vi "Move.vi"(0 "FSM.Edge in":refnum<class "FSM.Edge.lvclass">, 9 "delta":cluster{"X":dbl, "Y":dbl}) -> (4 "FSM.Edge out":refnum<class "FSM.Edge.lvclass">)   [LabVIEW 2020, in "FSM.Edge.lvclass"]
uses:
  FSM.Edge.lvclass
  FSM.Edge.lvclass/FSM.Edge.ctl
  FSM.Label/FSM.Label.lvclass
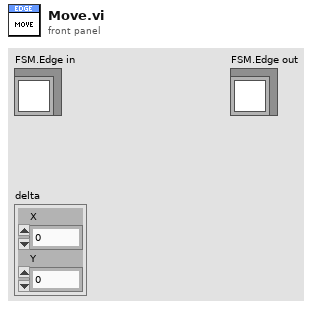
[diagram p1: front panel]
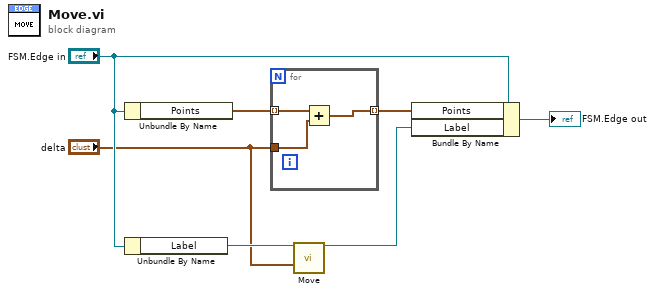
[diagram p0: block diagram]
diagram:
  n1 = Unbundle By Name("FSM.Edge in") -> ("Points"=w2:cluster{"x":i16, "y":i16}[])
  n2 = Unbundle By Name("FSM.Edge in") -> ("Label"=w4:refnum<class "FSM.Label.lvclass">)
  n3 = for {
    tunnel: "delta" -> [w10]
    tunnel: w2 -> [w9] mode=indexing
    tunnel: [w8] -> w1 mode=indexing
    n4 = Add(x=w9, y=w10) -> (x+y=w8:cluster{dbl, dbl})
  }
  n5 = call "Move.vi"("FSM.Label In"=w4, "delta"="delta") -> ("FSM.Label Out"=w5:refnum<class "FSM.Label.lvclass">)  [unwired: 13 in]
  n6 = Bundle By Name(cluster="FSM.Edge in", "Points"=w1, "Label"=w5) -> (→"FSM.Edge out":refnum<class "FSM.Edge.lvclass">)
